vi "RS232通訊-編碼.vi"(6 "排":enum16{"第一排", "第二排"}(ring), 8 "error in (no error)":errorcluster, 9 "線段":enum16{"左邊線段", "右邊線段"}(ring), 10 "Ring":u16(ring), 11 "量測值Array":dbl[](array[numeric])) -> (0 "error out":errorcluster, 3 "命令字串":string)   [LabVIEW 2013]
panel:
  out "Y座標":dbl
  out "Y座標":string="-20.000"
  out "命令Array":string[](array[string])
  # "參數"
  # "程式編號prog#"
  # "Block#"
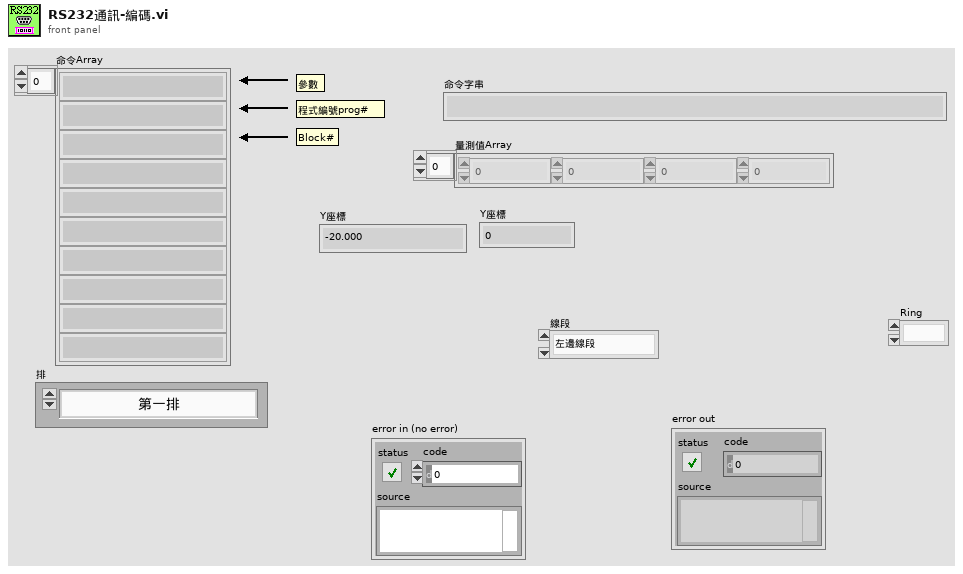
[diagram p1: front panel]
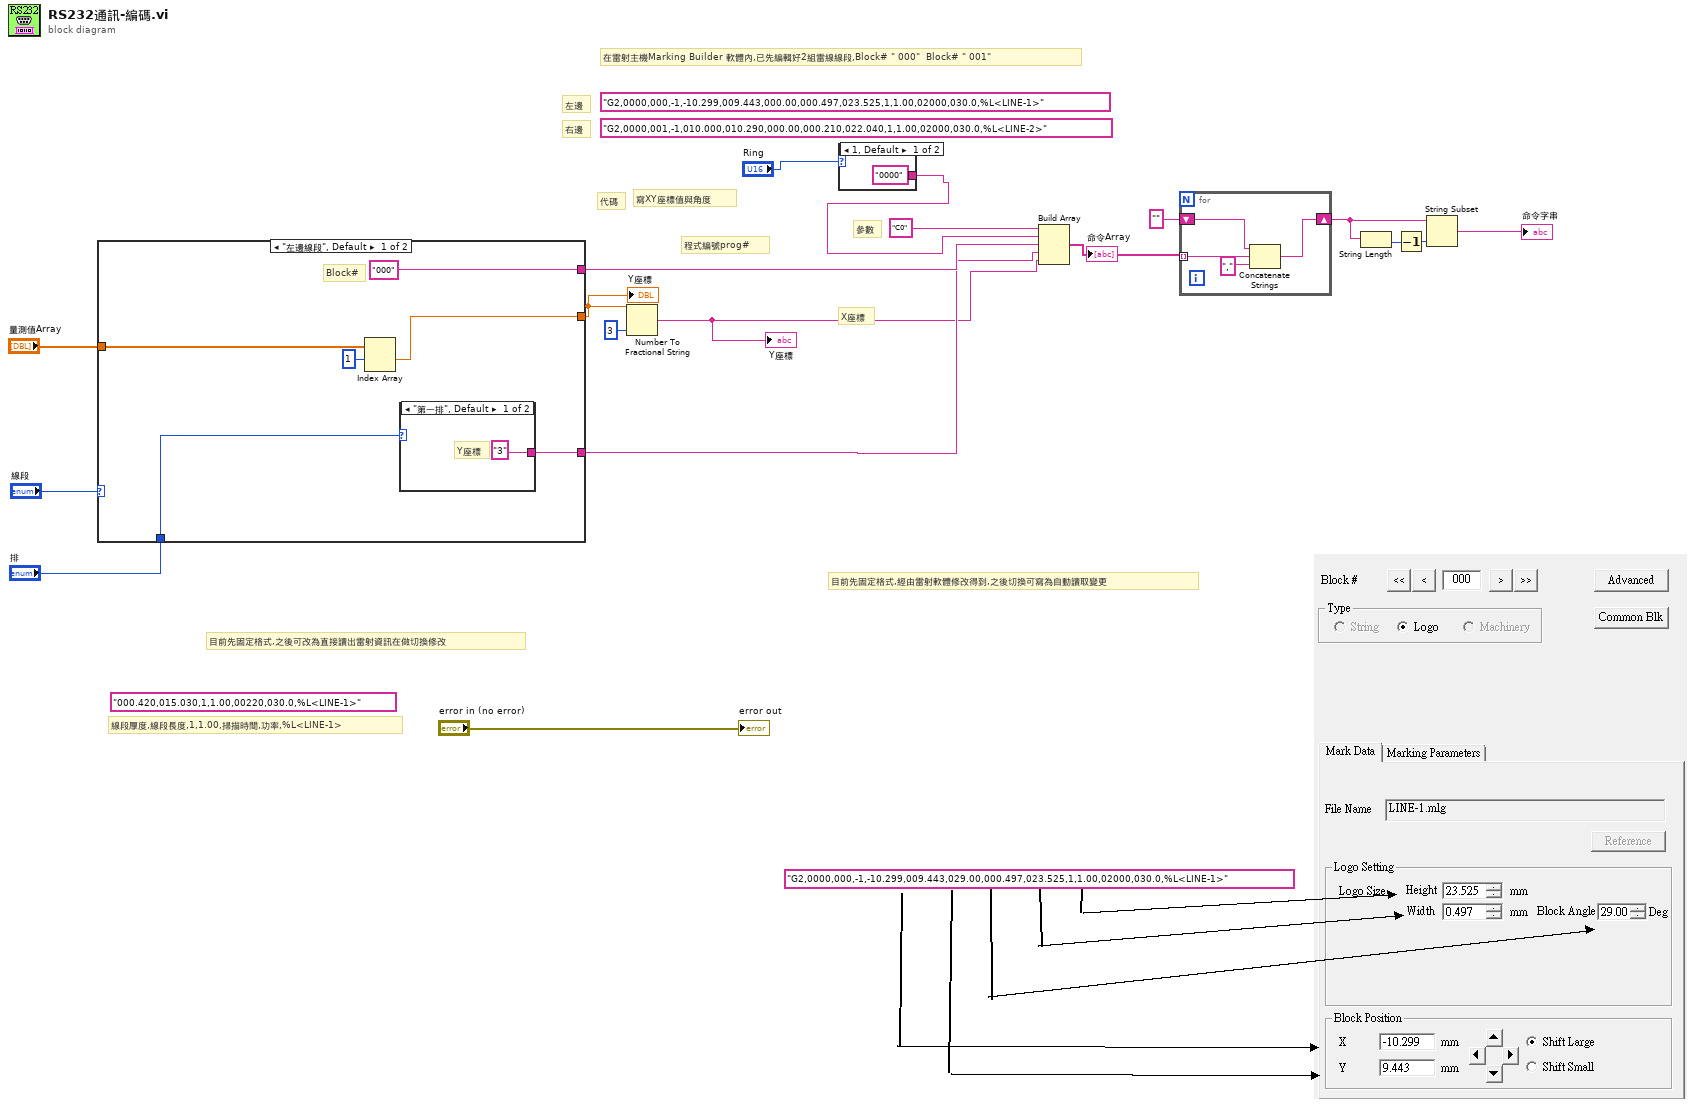
[diagram p0: block diagram]
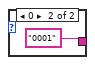
[diagram p2: hidden frame]
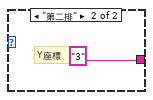
[diagram p3: hidden frame]
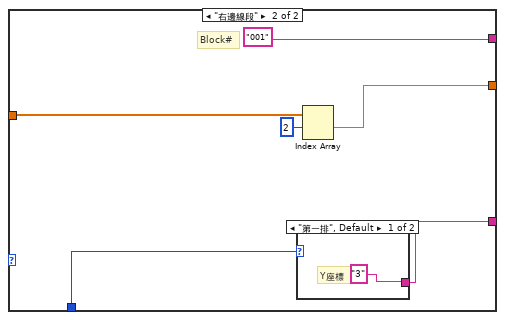
[diagram p4: hidden frame]
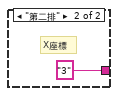
[diagram p5: hidden frame]
diagram:
  (unwired) "000.420,015.030,1,1.00,00220,030.0,%L<LINE-1>"
  (unwired) "G2,0000,000,-1,-10.299,009.443,029.00,000.497,023.525,1,1.00,02000,030.0,%L<LINE-1>"
  (unwired) "G2,0000,001,-1,010.000,010.290,000.00,000.210,022.040,1,1.00,02000,030.0,%L<LINE-2>"
  (unwired) "G2,0000,000,-1,-10.299,009.443,000.00,000.497,023.525,1,1.00,02000,030.0,%L<LINE-1>"
  # "線段厚度,線段長度,1,1.00,掃描時間,功率,%L<LINE-1>"
  # "目前先固定格式,經由雷射軟體修改得到,之後切換可寫為自動讀取變更"
  # "目前先固定格式,之後可改為直接讀出雷射資訊在做切換修改"
  # "代碼"
  # "右邊"
  # "左邊"
  # "在雷射主機Marking Builder 軟體內,已先編輯好2組雷線線段,Block# \" 000\"  Block# \" 001\""
  # "寫XY座標值與角度"
  # "X座標"
  # "程式編號prog#"
  # "參數"
  n1 = case shown="\"左邊線段\", Default" "線段" {
    tunnel: ["000" "001"] -> w8
    tunnel: "量測值Array" -> [w23 w30]
    tunnel: [w21 w29] -> w6
    tunnel: "排" -> [w20 w28]
    tunnel: [w19 w27] -> w4
    frame "左邊線段", Default {
      # "Block#"
      n2 = Index Array(array=w23, index #1=1 ("index")) -> (element #1=w21:dbl)  [unwired: 1 in, 1 out]
      n3 = case shown="\"第一排\", Default" w20 {
        tunnel: ["3" "3"] -> w19
        frame "第一排", Default {
          # "Y座標"
        }
        frame "第二排" {
          # "Y座標"
        }
      }
    }
    frame "右邊線段" {
      # "Block#"
      n4 = case shown="\"第一排\", Default" w28 {
        tunnel: ["3" "3"] -> w27
        frame "第一排", Default {
          # "Y座標"
        }
        frame "第二排" {
          # "X座標"
        }
      }
      n5 = Index Array(array=w30, index #1=2 ("index")) -> (element #1=w29:dbl)  [unwired: 1 in, 1 out]
    }
  }
  "Y座標" <- w6
  n6 = Number To Fractional String(number=w6, precision (6)=i16 3) -> (F-format string=w3:string)  [unwired: 2 in]
  "Y座標" <- w3
  n7 = case shown="1, Default" "Ring" {
    tunnel: ["0000" "0001"] -> w2
    frame 1, Default {
    }
    frame 0 {
    }
  }
  n8 = Build Array("C0", w2, w8, w4, w3) -> (w11:string[])
  "命令Array" <- w11
  n9 = for {
    tunnel: w11 -> [w38] mode=indexing
    shift-right: [w37] -> w15
    shift-left: "" -> [w39]
    n10 = Concatenate Strings(w39, w38, ",") -> (w37:string)
  }
  n11 = String Length(string=w15) -> (length=w16:i32)
  n12 = Decrement(x=w16) -> (x-1=w17:i32)
  n13 = String Subset(string=w15, length (rest)=w17) -> (substring=→"命令字串":string)  [unwired: 1 in]
  "error out" <- "error in (no error)"
